vi "Acquire.vi"(6 "Count In":i32, 8 "error in (no error)":errorcluster, 9 "Data Queue":refnum<queue>, 10 "APD Data Notifier":refnum<notifier>, 11 "HW Resources In":T1={"Data Source"=0, "Counter Configuration"={"DAQmx Task"="", "Counter(s)"="Dev2/ctr0", "samples per readout"=100}, "ADC Configuration"={"DAQmx Task"="", "Channel(s)"="Dev2/ctr0", "samples per readout"=100, "Sample Rate (s/s)"=100, "Max Voltage"=100.0, "Min Voltage"=100.0}} {"Data Source" items=["Counter", "ADC"]}) -> (0 "error out":errorcluster, 3 "HW Resources Out":T1={"Data Source"=0, "Counter Configuration"={"DAQmx Task"="", "Counter(s)"="Dev2/ctr0", "samples per readout"=100}, "ADC Configuration"={"DAQmx Task"="", "Channel(s)"="Dev2/ctr0", "samples per readout"=100, "Sample Rate (s/s)"=100, "Max Voltage"=100.0, "Min Voltage"=100.0}} {"Data Source" items=["Counter", "ADC"]}, 4 "Cout Out":i32)   [LabVIEW 2013, in "Acquisition.lvlib"]
doc: "Perform the acquisition. Replace the contents of this diagram with calls to acquisition hardware."
uses:
  Acquisition.lvlib
  Hardware Configuration.ctl
  Counter Configuration.ctl
  ADC/ADC Configuration.ctl
  APD Notifier Cluster.ctl
  <vilib>/DAQmx/read.llb/DAQmx Read (Counter 1D DBL 1Chan NSamp).vi
  <vilib>/DAQmx/read.llb/DAQmx Read (Analog 1D Wfm NChan NSamp).vi
  <resource>/objmgr/daqmx.rc
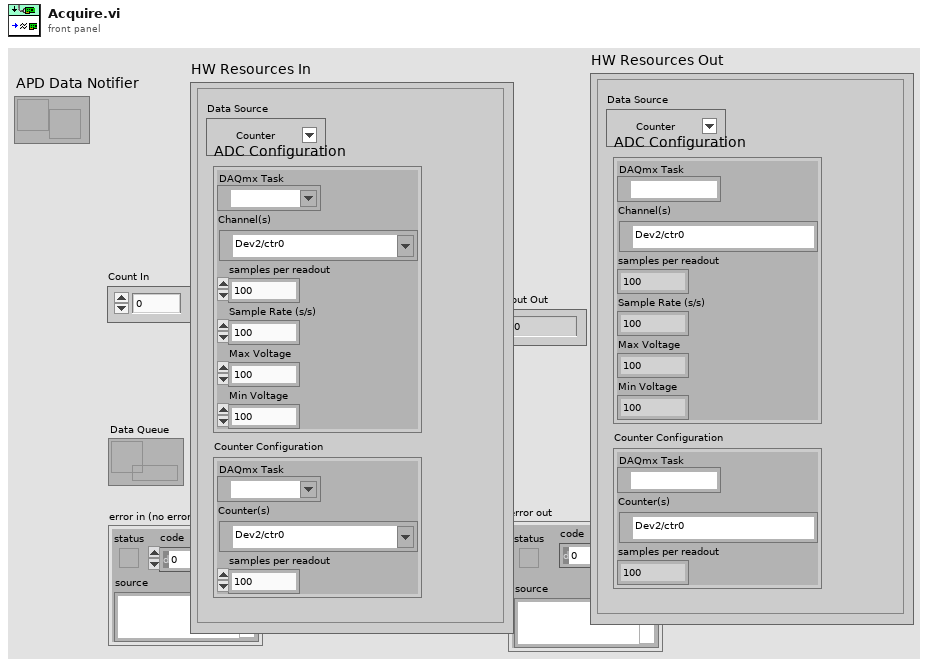
[diagram p1: front panel]
types:
  T1 = typedef "Acquisition.lvlib/Hardware Configuration.ctl" = cluster{"Data Source":u16, "Counter Configuration":T2, "ADC Configuration":T3}
  T2 = typedef "Acquisition.lvlib/Counter Configuration.ctl" = cluster{"DAQmx Task":refnum<k21>, "Counter(s)":tag, "samples per readout":i32}
  T3 = typedef "Acquisition.lvlib/ADC Configuration.ctl" = cluster{"DAQmx Task":refnum<k21>, "Channel(s)":tag, "samples per readout":i32, "Sample Rate (s/s)":i32, "Max Voltage":dbl, "Min Voltage":dbl}
  T4 = typedef "Acquisition.lvlib/APD Notifier Cluster.ctl" = cluster{"data":dbl[][], "t0":i32}
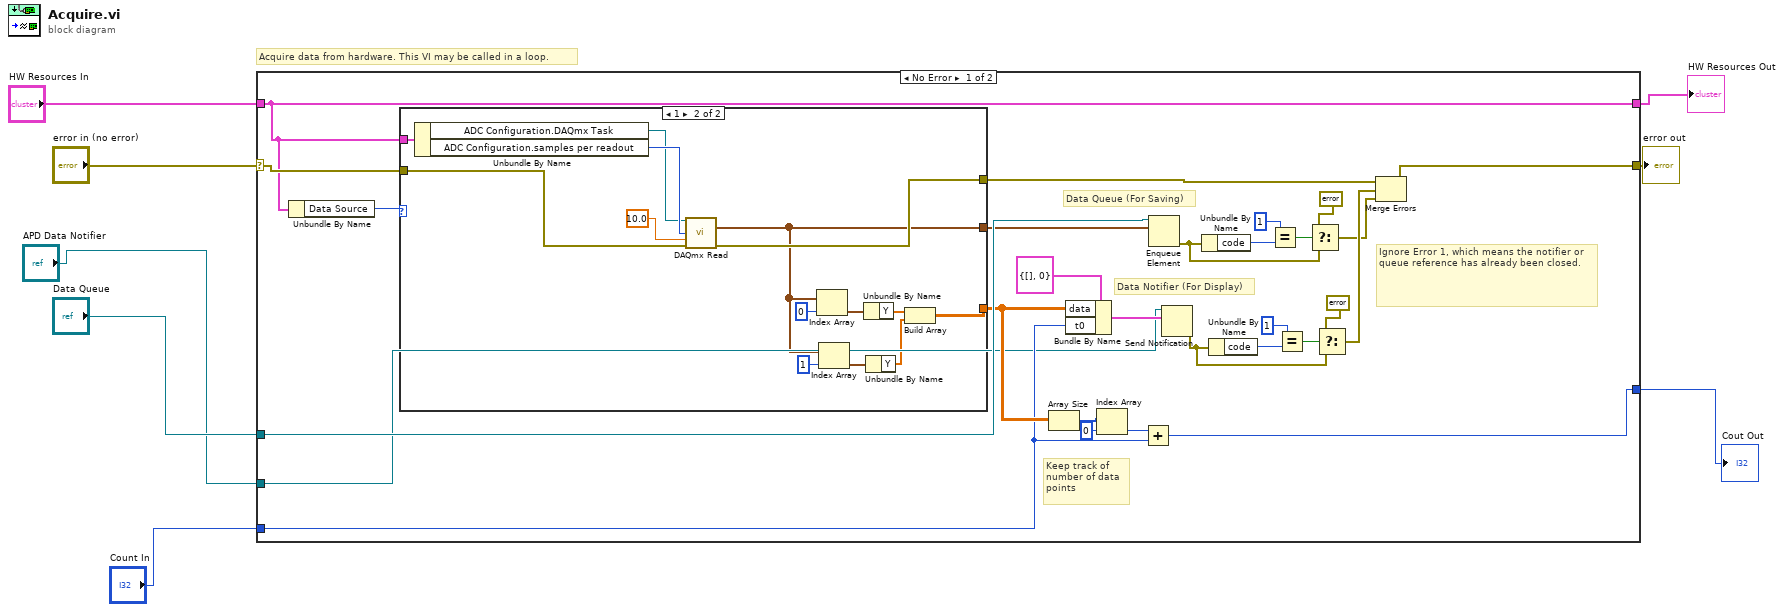
[diagram p0: block diagram]
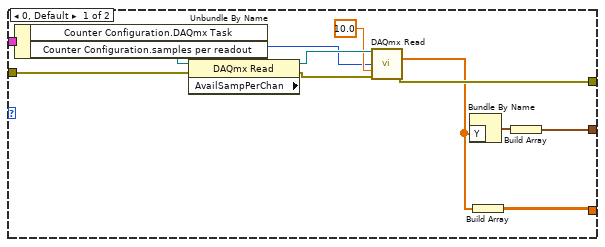
[diagram p2: hidden frame]
diagram:
  # "Acquire data from hardware. This VI may be called in a loop."
  n1 = case shown="No Error" "error in (no error)" {
    selector: "error in (no error)" -> [w22 w64]
    tunnel: [w36 w64] -> w7
    tunnel: "HW Resources In" -> [w14 w65]
    tunnel: [w14 w65] -> w3
    tunnel: "Data Queue" -> [w24 _]
    tunnel: "APD Data Notifier" -> [w12 _]
    tunnel: "Count In" -> [w15 w63]
    tunnel: [w19 w63] -> w4
    frame No Error {
      # "Data Notifier (For Display)"
      # "Data Queue (For Saving)"
      # "Keep track of\nnumber of data\npoints"
      # "Ignore Error 1, which means the notifier or queue reference has already been closed."
      n2 = Unbundle By Name(w14) -> ("Data Source"=w13:u16)
      n3 = case shown="1" w13 {
        tunnel: w14 -> [w48 w62]
        tunnel: [w47 w61] -> w23
        tunnel: w22 -> [w45 w57]
        tunnel: [w39 w50] -> w21
        tunnel: [w37 w53] -> w16
        frame 0, Default {
          n4 = Unbundle By Name(w48) -> ("Counter Configuration.DAQmx Task"=w46:refnum<k21>, "Counter Configuration.samples per readout"=w42:i32)
          n5 = property class="DAQmx Read" props=["AvailSampPerChan"](reference=w46, error in=w45) -> (reference out=w44:refnum<k21>, error out=w41:errorcluster)  [unwired: 1 out]
          n6 = call-poly <vilib>:"DAQmx Read.vi"("task/channels in"=w44, "number of samples per channel"=w42, "timeout"=10.0, "error in"=w41) -> ("data"=w38:dbl[], "error out"=w47:errorcluster)  [unwired: 9 in, 1 out]
          n7 = Bundle By Name("Y"=w38) -> (w40:waveform(dbl))  [unwired: 1 in]
          n8 = Build Array(w38) -> (w37:dbl[][])
          n9 = Build Array(w40) -> (w39:waveform(dbl)[])
        }
        frame 1 {
          n10 = Unbundle By Name(w62) -> ("ADC Configuration.DAQmx Task"=w58:refnum<k21>, "ADC Configuration.samples per readout"=w59:i32)
          n11 = call-poly <vilib>:"DAQmx Read.vi"("task/channels in"=w58, "number of samples per channel"=w59, "timeout"=10.0, "error in"=w57) -> ("data"=w50:waveform(dbl)[], "error out"=w61:errorcluster)  [unwired: 9 in, 1 out]
          n12 = Index Array(array=w50, index=0) -> (element=w55:waveform(dbl))
          n13 = Index Array(array=w50, index=1) -> (element=w51:waveform(dbl))
          n14 = Unbundle By Name(w55) -> ("Y"=w54:dbl[])
          n15 = Unbundle By Name(w51) -> ("Y"=w49:dbl[])
          n16 = Build Array(w54, w49) -> (w53:dbl[][])
        }
      }
      n17 = Array Size(array=w16) -> (size(s)=w11:i32[])
      n18 = Bundle By Name(cluster=T4 {"data"=[], "t0"=0} ("APD Data Notifier Cluster"), "data"=w16, "t0"=w15) -> (w18:T4)
      n19 = Index Array(array=w11, index=0) -> (element=w9:i32)
      n20 = Add(x=w9, y=w15) -> (x+y=w19:i32)
      n21 = Enqueue Element(queue=w24, element=w21) -> (error out=w29:errorcluster)  [unwired: 2 in, 2 out]
      n22 = Send Notification(notification=w18, notifier=w12) -> (error out=w20:errorcluster)  [unwired: 1 in, 1 out]
      n23 = Unbundle By Name(w29) -> ("code"=w26:i32)
      n24 = Unbundle By Name(w20) -> ("code"=w35:i32)
      n25 = Equal?(x=1, y=w26) -> (x = y?=w28:bool)
      n26 = Equal?(x=1, y=w35) -> (x = y?=w33:bool)
      n27 = Select(t=errorcluster {"status"=FALSE, "code"=0, "source"=""} ("error constant"), s=w28, f=w29) -> (s? t:f=w25:errorcluster)
      n28 = Select(t=errorcluster {"status"=FALSE, "code"=0, "source"=""} ("error constant"), s=w33, f=w20) -> (s? t:f=w32:errorcluster)
      n29 = Merge Errors(w23, w32, w25) -> (w36:errorcluster)
    }
    frame Error {
    }
  }
  "error out" <- w7
  "Cout Out" <- w4
  "HW Resources Out" <- w3
